vi "Trajectory Enabled.vi"() -> ()   [LabVIEW 2019]
panel:
  in  "Trajectory Enabled":bool
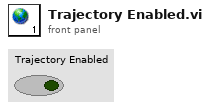
[diagram p1: front panel]
diagram:
